vi "changeScale.vi"(8 "error in (no error)":errorcluster, 11 "PixelflySettings in":refnum<class "PixelflySettings.lvclass">) -> (0 "error out":errorcluster, 3 "PixelflySettings out":refnum<class "PixelflySettings.lvclass">)   [LabVIEW 2009, in "Tools.lvlib" / "Settings.lvlib" / "PixelflySettings.lvclass"]
uses:
  PixelflySettings.lvclass
  PixelflySettings.lvclass/PixelflySettings.ctl
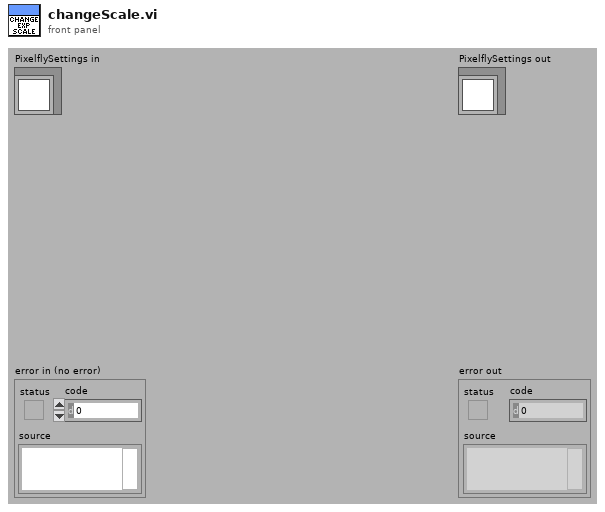
[diagram p1: front panel]
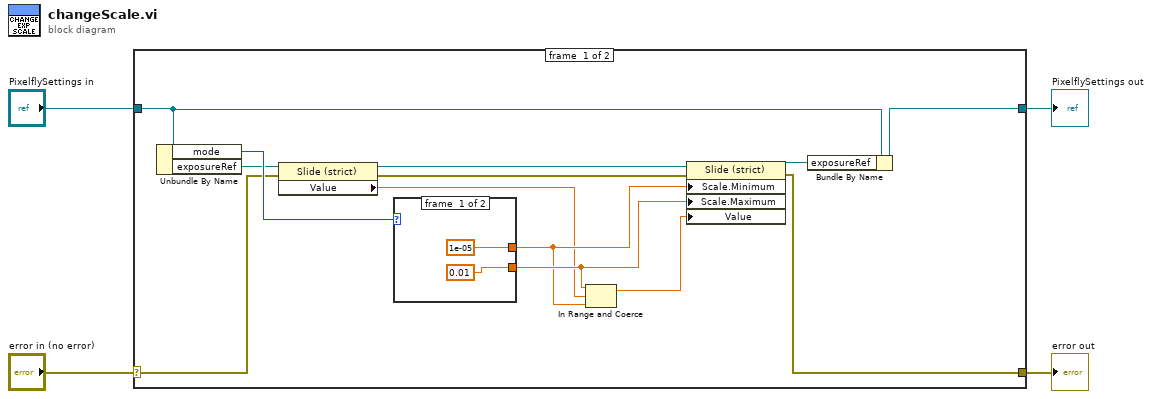
[diagram p0: block diagram]
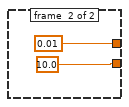
[diagram p2: hidden frame]
diagram:
  n1 = case shown="No Error" "error in (no error)" {
    selector: "error in (no error)" -> [w11 w23]
    tunnel: [w17 w23] -> w3
    tunnel: [w13 w22] -> w1
    tunnel: "PixelflySettings in" -> [w14 w22]
    frame #0 {
      n2 = Unbundle By Name(w14) -> ("mode"=w16:u16, "exposureRef"=w12:refnum<vi>)
      n3 = property class="Slide (strict)"(reference=w12, error in=w11) -> (reference out=w9:refnum<vi>, error out=w10:errorcluster, "Value"=w6:dbl)
      n4 = case shown="0, Default" w16 {
        tunnel: [1e-05 0.01] -> w7
        tunnel: [0.01 10.0] -> w8
        frame #0 {
        }
        frame #1 {
        }
      }
      n5 = In Range and Coerce(upper limit=w8, x=w6, lower limit=w7) -> (coerced(x)=w5:dbl)  [unwired: 1 out]
      n6 = property class="Slide (strict)"(reference=w9, error in=w10, "Scale.Minimum"=w7, "Scale.Maximum"=w8, "Value"=w5) -> (reference out=w15:refnum<vi>, error out=w17:errorcluster)
      n7 = Bundle By Name(cluster=w14, "exposureRef"=w15) -> (w13:refnum<class "PixelflySettings.lvclass">)
    }
    frame #1 {
    }
  }
  "error out" <- w3
  "PixelflySettings out" <- w1
